vi "Climb_Motors.vi"(4 "Driver - Right Thumb":bool, 5 "Driver - Left Middle":bool, 6 "Driver - Left Thumb":bool, 7 "Driver - Right Middle":bool, 8 "Driver - Trigger":bool, 9 "Driver - Left Top left":bool, 10 "Driver - Right Top Right":bool) -> ()   [LabVIEW 2020]
uses:
  <vilib>/Rock Robotics/WPI/ThirdParty/Phoenix-LabVIEW/Motor Controller/Controls/CTRE_Phoenix_MotorControl_ControlMode.ctl
  <vilib>/Rock Robotics/Network Tables/NT Read String.vi
panel:
  in  "Traversal 1":dbl
  in  "Traversal 2":dbl
  in  "High 1":dbl
  in  "High 2":dbl
  in  "Mid 1":dbl=377500.0
  in  "Mid 2":dbl=377500.0
  in  "Low 1":dbl=150000.0
  in  "Low 2":dbl=150000.0
  in  "Low 4":dbl=150000.0
  in  "Low 3":dbl=150000.0
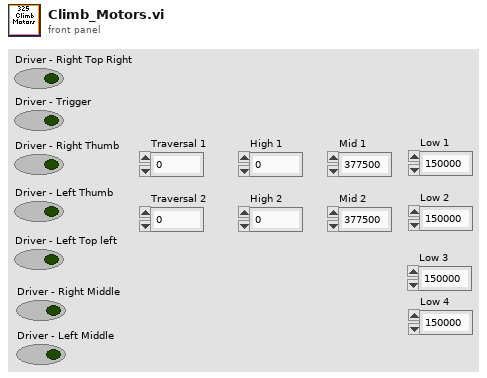
[diagram p1: front panel]
types:
  T1 = typedef "WPI_MotorControlDeviceRef.ctl" = cluster{"DeviceStatus":errorcluster, "Type":T2, "PWM":cluster{"PWM Channel":T3, "DeadBand":T4}, "CAN":cluster{"Device Number":u8, "SetOutput VI Ref":variant, "GetOutput VI Ref":variant, "Enable VI Ref":variant, "Disable VI Ref":variant, "Data":variant}, "Invert":bool, "DIO PWM":cluster{"PWM \"Enable\" Channel":T3, "DIOChannel":T5, "PWM Rate":dbl}}
  T2 = typedef "WPI_MotorControlType.ctl" = enum16{"PWM", "CAN", "DIO PWM"}
  T3 = typedef "FPGA_DIOPWMChannel.ctl" = enum8{"PWM 0", "PWM 1", "PWM 2", "PWM 3", "PWM 4", "PWM 5", "PWM 6", "PWM 7", "PWM 8", "PWM 9", "PWM MXP 0", "PWM MXP 1", "PWM MXP 2", "PWM MXP 3", "PWM MXP 4", "PWM MXP 5", "PWM MXP 6", "PWM MXP 7", "PWM MXP 8", "PWM MXP 9", "Invalid"}
  T4 = typedef "WPI_PWMDeadband.ctl" = cluster{"Name":string, "maxPositivePwm":i32, "minPositivePwm":i32, "centerPwm":i32, "maxNegativePwm":i32, "minNegativePwm":i32, "angularRange":u16}
  T5 = typedef "FPGA_DIOChannel.ctl" = enum8{"DIO 0", "DIO 1", "DIO 2", "DIO 3", "DIO 4", "DIO 5", "DIO 6", "DIO 7", "DIO 8", "DIO 9", "DIO MXP 0", "DIO MXP 1", "DIO MXP 2", "DIO MXP 3", "DIO MXP 4", "DIO MXP 5", "DIO MXP 6", "DIO MXP 7", "DIO MXP 8", "DIO MXP 9", "DIO MXP 10", "DIO MXP 11", "DIO MXP 12", "DIO MXP 13", "DIO MXP 14", "DIO MXP 15", "SPI Port CS1", "SPI Port CS2", "SPI Port CS3", "SPI Port MISO", "SPI Port MOSI", "Invalid"}
  T6 = typedef "CTRE_Phoenix_MotorControl_ControlMode.ctl" = u16
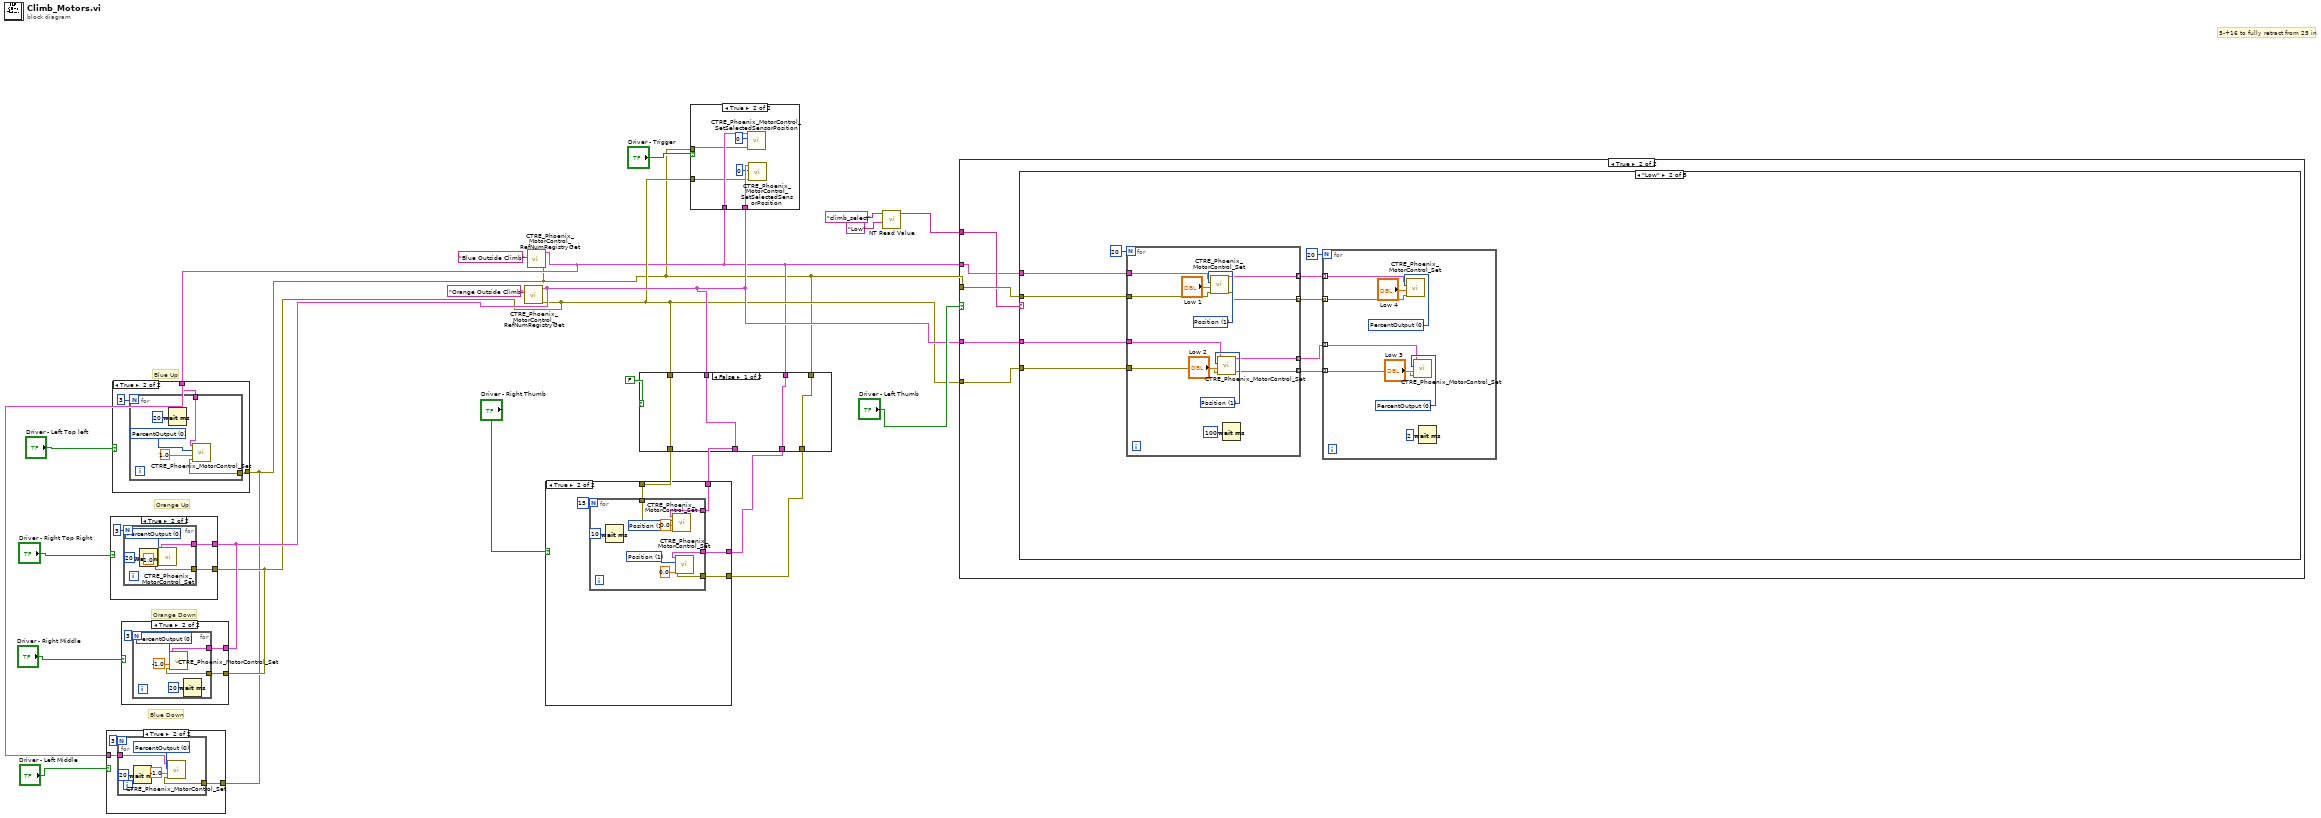
[diagram p0: block diagram]
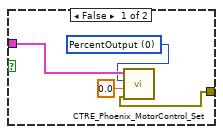
[diagram p2: hidden frame]
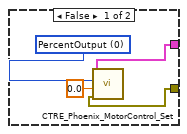
[diagram p3: hidden frame]
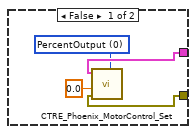
[diagram p4: hidden frame]
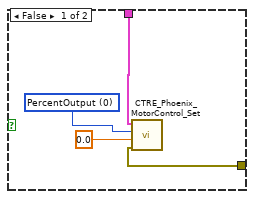
[diagram p5: hidden frame]
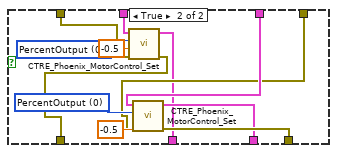
[diagram p6: hidden frame]
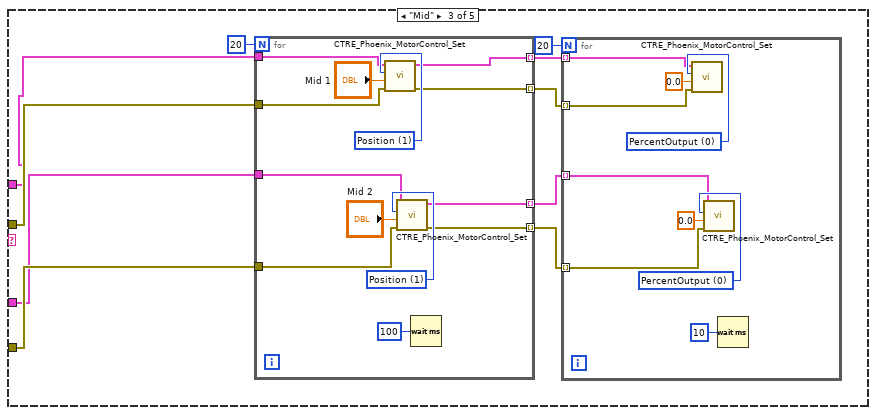
[diagram p10: hidden frame]
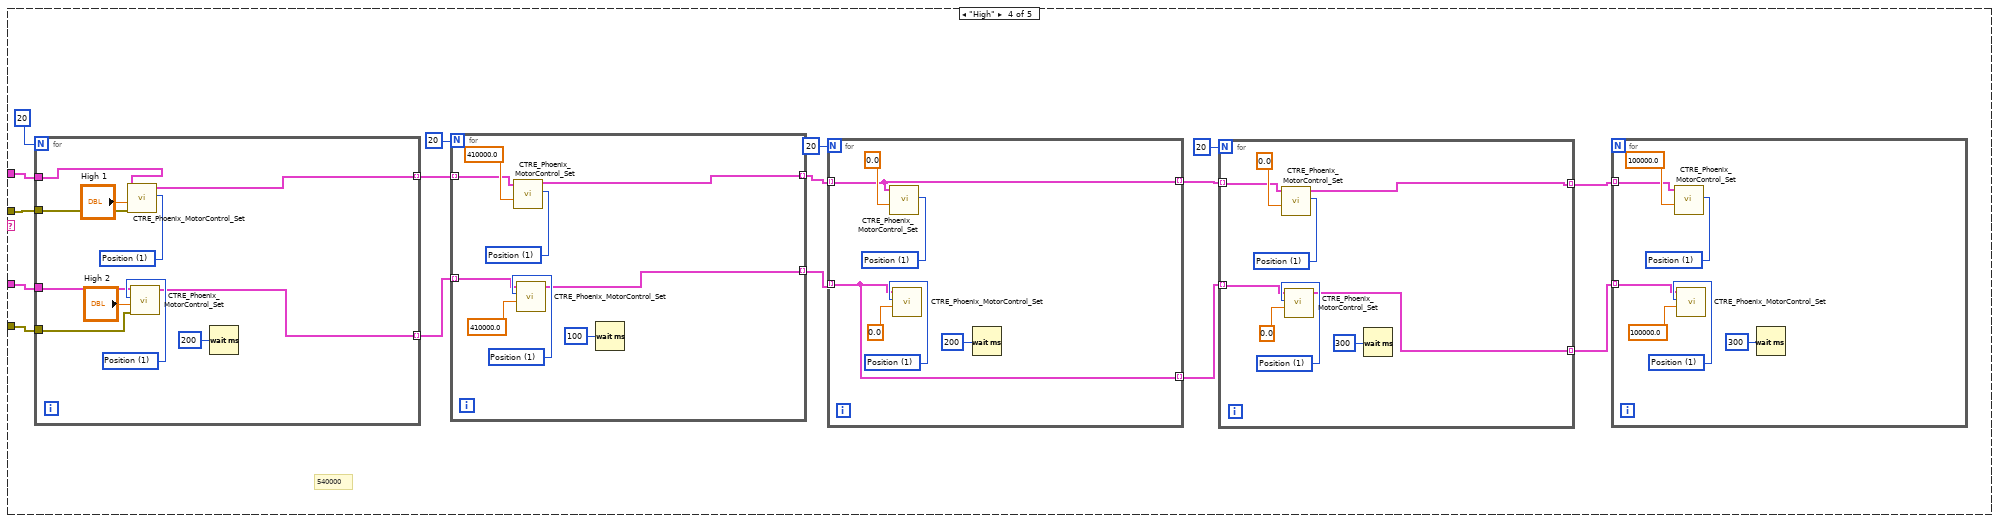
[diagram p11: hidden frame]
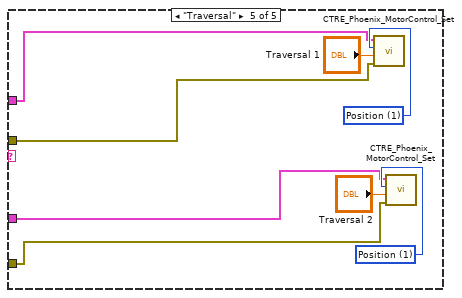
[diagram p12: hidden frame]
diagram:
  # "Blue Down"
  # "Orange Down"
  # "Orange Up"
  # "Blue Up"
  # "5-+16 to fully retract from 25 in"
  n1 = call <vilib>:"CTRE_Phoenix_MotorControl_RefNumRegistryGet.vi"("refnum name"="Orange Outside Climb") -> ("error out"=w4:errorcluster, "PhoenixMotorControlDevRef"=w5:T1)  [unwired: 9 in]
  n2 = case shown="True" "Driver - Right Top Right" {
    tunnel: w5 -> [w23 w28]
    tunnel: w4 -> [w24 w27]
    frame False {
      w22 = T6 0 items=["PercentOutput"=0, "Position"=1, "Velocity"=2, "Current"=3, "Follower"=5, "MotionProfile"=6, "MotionMagic"=7, "MotionProfileArc"=10, "Disabled"=15] ("Control Mode")
      n3 = call <vilib>:"CTRE_Phoenix_MotorControl_Set.vi"("error in (no error)"=w24, "Output"=0.0, "Control Mode"=w22, "PhoenixMotorControlDevRef"=w23) -> ()  [unwired: 6 in, 2 out]
    }
    frame True {
      n4 = for {
        N: 3 -> [_]
        tunnel: w28 -> [w31]
        tunnel: w27 -> [w30]
        w33 = T6 0 items=["PercentOutput"=0, "Position"=1, "Velocity"=2, "Current"=3, "Follower"=5, "MotionProfile"=6, "MotionMagic"=7, "MotionProfileArc"=10, "Disabled"=15] ("Control Mode")
        n5 = Wait (ms)(milliseconds to wait=u32 20) -> ()  [unwired: 1 out]
        n6 = call <vilib>:"CTRE_Phoenix_MotorControl_Set.vi"("error in (no error)"=w30, "Output"=1.0, "Control Mode"=w33, "PhoenixMotorControlDevRef"=w31) -> ()  [unwired: 6 in, 2 out]
      }
    }
  }
  n7 = case shown="True" "Driver - Right Middle" {
    tunnel: w5 -> [w35 w40]
    tunnel: w4 -> [w36 w39]
    frame False {
      w34 = T6 0 items=["PercentOutput"=0, "Position"=1, "Velocity"=2, "Current"=3, "Follower"=5, "MotionProfile"=6, "MotionMagic"=7, "MotionProfileArc"=10, "Disabled"=15] ("Control Mode")
      n8 = call <vilib>:"CTRE_Phoenix_MotorControl_Set.vi"("error in (no error)"=w36, "Output"=0.0, "Control Mode"=w34, "PhoenixMotorControlDevRef"=w35) -> ()  [unwired: 6 in, 2 out]
    }
    frame True {
      n9 = for {
        N: 3 -> [_]
        tunnel: w40 -> [w43]
        tunnel: w39 -> [w42]
        w45 = T6 0 items=["PercentOutput"=0, "Position"=1, "Velocity"=2, "Current"=3, "Follower"=5, "MotionProfile"=6, "MotionMagic"=7, "MotionProfileArc"=10, "Disabled"=15] ("Control Mode")
        n10 = call <vilib>:"CTRE_Phoenix_MotorControl_Set.vi"("error in (no error)"=w42, "Output"=-1.0, "Control Mode"=w45, "PhoenixMotorControlDevRef"=w43) -> ()  [unwired: 6 in, 2 out]
        n11 = Wait (ms)(milliseconds to wait=u32 20) -> ()  [unwired: 1 out]
      }
    }
  }
  n12 = call <vilib>:"CTRE_Phoenix_MotorControl_RefNumRegistryGet.vi"("refnum name"="Blue Outside Climb") -> ("error out"=w2:errorcluster, "PhoenixMotorControlDevRef"=w3:T1)  [unwired: 9 in]
  n13 = case shown="True" "Driver - Left Middle" {
    tunnel: w3 -> [w47 w52]
    tunnel: w2 -> [w48 w51]
    frame False {
      w46 = T6 0 items=["PercentOutput"=0, "Position"=1, "Velocity"=2, "Current"=3, "Follower"=5, "MotionProfile"=6, "MotionMagic"=7, "MotionProfileArc"=10, "Disabled"=15] ("Control Mode")
      n14 = call <vilib>:"CTRE_Phoenix_MotorControl_Set.vi"("error in (no error)"=w48, "Output"=0.0, "Control Mode"=w46, "PhoenixMotorControlDevRef"=w47) -> ()  [unwired: 6 in, 2 out]
    }
    frame True {
      n15 = for {
        N: 3 -> [_]
        tunnel: w52 -> [w55]
        tunnel: w51 -> [w54]
        w57 = T6 0 items=["PercentOutput"=0, "Position"=1, "Velocity"=2, "Current"=3, "Follower"=5, "MotionProfile"=6, "MotionMagic"=7, "MotionProfileArc"=10, "Disabled"=15] ("Control Mode")
        n16 = Wait (ms)(milliseconds to wait=u32 20) -> ()  [unwired: 1 out]
        n17 = call <vilib>:"CTRE_Phoenix_MotorControl_Set.vi"("error in (no error)"=w54, "Output"=-1.0, "Control Mode"=w57, "PhoenixMotorControlDevRef"=w55) -> ()  [unwired: 6 in, 2 out]
      }
    }
  }
  n18 = case shown="True" "Driver - Left Top left" {
    tunnel: w3 -> [w58 w64]
    tunnel: w2 -> [w59 w63]
    frame False {
      w60 = T6 0 items=["PercentOutput"=0, "Position"=1, "Velocity"=2, "Current"=3, "Follower"=5, "MotionProfile"=6, "MotionMagic"=7, "MotionProfileArc"=10, "Disabled"=15] ("Control Mode")
      n19 = call <vilib>:"CTRE_Phoenix_MotorControl_Set.vi"("error in (no error)"=w59, "Output"=0.0, "Control Mode"=w60, "PhoenixMotorControlDevRef"=w58) -> ()  [unwired: 6 in, 2 out]
    }
    frame True {
      n20 = for {
        N: 3 -> [_]
        tunnel: w64 -> [w67]
        tunnel: w63 -> [w66]
        w68 = T6 0 items=["PercentOutput"=0, "Position"=1, "Velocity"=2, "Current"=3, "Follower"=5, "MotionProfile"=6, "MotionMagic"=7, "MotionProfileArc"=10, "Disabled"=15] ("Control Mode")
        n21 = Wait (ms)(milliseconds to wait=u32 20) -> ()  [unwired: 1 out]
        n22 = call <vilib>:"CTRE_Phoenix_MotorControl_Set.vi"("error in (no error)"=w66, "Output"=1.0, "Control Mode"=w68, "PhoenixMotorControlDevRef"=w67) -> ()  [unwired: 6 in, 2 out]
      }
    }
  }
  n23 = case shown="False" FALSE {
    tunnel: w4 -> [w73 w80]
    tunnel: [w73 w74] -> w13
    tunnel: w5 -> [w72 w81]
    tunnel: [w72 w75] -> w12
    tunnel: [w71 w76] -> w11
    tunnel: w3 -> [w71 w79]
    tunnel: [w70 w77] -> w10
    tunnel: w2 -> [w70 w78]
    frame False {
    }
    frame True {
      w84 = T6 0 items=["PercentOutput"=0, "Position"=1, "Velocity"=2, "Current"=3, "Follower"=5, "MotionProfile"=6, "MotionMagic"=7, "MotionProfileArc"=10, "Disabled"=15] ("Control Mode")
      w85 = T6 0 items=["PercentOutput"=0, "Position"=1, "Velocity"=2, "Current"=3, "Follower"=5, "MotionProfile"=6, "MotionMagic"=7, "MotionProfileArc"=10, "Disabled"=15] ("Control Mode")
      n24 = call <vilib>:"CTRE_Phoenix_MotorControl_Set.vi"("error in (no error)"=w80, "Output"=-0.5, "Control Mode"=w84, "PhoenixMotorControlDevRef"=w81) -> ("error out"=w74:errorcluster, "PhoenixMotorControlDevRef"=w75:T1)  [unwired: 6 in]
      n25 = call <vilib>:"CTRE_Phoenix_MotorControl_Set.vi"("error in (no error)"=w78, "Output"=-0.5, "Control Mode"=w85, "PhoenixMotorControlDevRef"=w79) -> ("error out"=w77:errorcluster, "PhoenixMotorControlDevRef"=w76:T1)  [unwired: 6 in]
    }
  }
  n26 = case shown="True" "Driver - Right Thumb" {
    tunnel: w12 -> [_ w90]
    tunnel: w13 -> [_ w89]
    tunnel: w11 -> [_ w88]
    tunnel: w10 -> [_ w87]
    frame False {
    }
    frame True {
      n27 = for {
        N: 15 -> [_]
        tunnel: w90 -> [w95]
        tunnel: w89 -> [w94]
        tunnel: w88 -> [w93]
        tunnel: w87 -> [w92]
        w98 = T6 1 items=["PercentOutput"=0, "Position"=1, "Velocity"=2, "Current"=3, "Follower"=5, "MotionProfile"=6, "MotionMagic"=7, "MotionProfileArc"=10, "Disabled"=15] ("Control Mode")
        w99 = T6 1 items=["PercentOutput"=0, "Position"=1, "Velocity"=2, "Current"=3, "Follower"=5, "MotionProfile"=6, "MotionMagic"=7, "MotionProfileArc"=10, "Disabled"=15] ("Control Mode")
        n28 = Wait (ms)(milliseconds to wait=u32 10) -> ()  [unwired: 1 out]
        n29 = call <vilib>:"CTRE_Phoenix_MotorControl_Set.vi"("error in (no error)"=w94, "Output"=0.0, "Control Mode"=w98, "PhoenixMotorControlDevRef"=w95) -> ()  [unwired: 6 in, 2 out]
        n30 = call <vilib>:"CTRE_Phoenix_MotorControl_Set.vi"("error in (no error)"=w92, "Output"=0.0, "Control Mode"=w99, "PhoenixMotorControlDevRef"=w93) -> ()  [unwired: 6 in, 2 out]
      }
    }
  }
  n31 = case shown="True" "Driver - Trigger" {
    tunnel: w3 -> [_ w105]
    tunnel: w2 -> [_ w104]
    tunnel: w5 -> [_ w103]
    tunnel: w4 -> [_ w102]
    frame False {
    }
    frame True {
      n32 = call <vilib>:"CTRE_Phoenix_MotorControl_SetSelectedSensorPosition.vi"("error in (no error)"=w104, "New Sensor Position"=0, "PhoenixMotorControlDevRef"=w105) -> ()  [unwired: 7 in, 2 out]
      n33 = call <vilib>:"CTRE_Phoenix_MotorControl_SetSelectedSensorPosition.vi"("error in (no error)"=w102, "New Sensor Position"=0, "PhoenixMotorControlDevRef"=w103) -> ()  [unwired: 7 in, 2 out]
    }
  }
  n34 = call-poly <vilib>:"NT Read Value.vi"("Default Value"="Low", "Name"="climb_select") -> ("String"=w16:string)  [unwired: 8 in, 1 out]
  n35 = case shown="True" "Driver - Left Thumb" {
    tunnel: w3 -> [_ w106]
    tunnel: w2 -> [_ w110]
    tunnel: w5 -> [_ w109]
    tunnel: w4 -> [_ w108]
    tunnel: w16 -> [_ w107]
    frame False {
    }
    frame True {
      n36 = case shown="\"Low\"" w107 {
        tunnel: w110 -> [_ w120 w152 w190 w237]
        tunnel: w109 -> [_ w119 w150 w189 w236]
        tunnel: w108 -> [_ w118 w151 w188 w235]
        tunnel: w106 -> [_ w117 w149 w187 w234]
        frame Default {
        }
        frame "Low" {
          n37 = for {
            N: 20 -> [_]
            tunnel: w120 -> [w140]
            tunnel: w119 -> [w137]
            tunnel: w118 -> [w136]
            tunnel: w117 -> [w135]
            tunnel: [w133] -> w115 mode=indexing
            tunnel: [w132] -> w114 mode=indexing
            tunnel: [w131] -> w113 mode=indexing
            tunnel: [w130] -> w112 mode=indexing
            w138 = T6 1 items=["PercentOutput"=0, "Position"=1, "Velocity"=2, "Current"=3, "Follower"=5, "MotionProfile"=6, "MotionMagic"=7, "MotionProfileArc"=10, "Disabled"=15] ("Control Mode")
            w141 = T6 1 items=["PercentOutput"=0, "Position"=1, "Velocity"=2, "Current"=3, "Follower"=5, "MotionProfile"=6, "MotionMagic"=7, "MotionProfileArc"=10, "Disabled"=15] ("Control Mode")
            n38 = call <vilib>:"CTRE_Phoenix_MotorControl_Set.vi"("error in (no error)"=w140, "Output"="Low 1", "Control Mode"=w141, "PhoenixMotorControlDevRef"=w135) -> ("error out"=w132:errorcluster, "PhoenixMotorControlDevRef"=w133:T1)  [unwired: 6 in]
            n39 = call <vilib>:"CTRE_Phoenix_MotorControl_Set.vi"("error in (no error)"=w136, "Output"="Low 2", "Control Mode"=w138, "PhoenixMotorControlDevRef"=w137) -> ("error out"=w130:errorcluster, "PhoenixMotorControlDevRef"=w131:T1)  [unwired: 6 in]
            n40 = Wait (ms)(milliseconds to wait=u32 100) -> ()  [unwired: 1 out]
          }
          n41 = for {
            N: 20 -> [_]
            tunnel: w114 -> [w127] mode=indexing
            tunnel: w113 -> [w124] mode=indexing
            tunnel: w112 -> [w123] mode=indexing
            tunnel: w115 -> [w122] mode=indexing
            w125 = T6 0 items=["PercentOutput"=0, "Position"=1, "Velocity"=2, "Current"=3, "Follower"=5, "MotionProfile"=6, "MotionMagic"=7, "MotionProfileArc"=10, "Disabled"=15] ("Control Mode")
            w128 = T6 0 items=["PercentOutput"=0, "Position"=1, "Velocity"=2, "Current"=3, "Follower"=5, "MotionProfile"=6, "MotionMagic"=7, "MotionProfileArc"=10, "Disabled"=15] ("Control Mode")
            n42 = call <vilib>:"CTRE_Phoenix_MotorControl_Set.vi"("error in (no error)"=w127, "Output"="Low 4", "Control Mode"=w128, "PhoenixMotorControlDevRef"=w122) -> ()  [unwired: 6 in, 2 out]
            n43 = call <vilib>:"CTRE_Phoenix_MotorControl_Set.vi"("error in (no error)"=w123, "Output"="Low 3", "Control Mode"=w125, "PhoenixMotorControlDevRef"=w124) -> ()  [unwired: 6 in, 2 out]
            n44 = Wait (ms)(milliseconds to wait=u32 2) -> ()  [unwired: 1 out]
          }
        }
        frame "Mid" {
          n45 = for {
            N: 20 -> [_]
            tunnel: w152 -> [w170]
            tunnel: w151 -> [w169]
            tunnel: w150 -> [w168]
            tunnel: w149 -> [w167]
            tunnel: [w165] -> w147 mode=indexing
            tunnel: [w164] -> w146 mode=indexing
            tunnel: [w163] -> w145 mode=indexing
            tunnel: [w162] -> w144 mode=indexing
            w171 = T6 1 items=["PercentOutput"=0, "Position"=1, "Velocity"=2, "Current"=3, "Follower"=5, "MotionProfile"=6, "MotionMagic"=7, "MotionProfileArc"=10, "Disabled"=15] ("Control Mode")
            w173 = T6 1 items=["PercentOutput"=0, "Position"=1, "Velocity"=2, "Current"=3, "Follower"=5, "MotionProfile"=6, "MotionMagic"=7, "MotionProfileArc"=10, "Disabled"=15] ("Control Mode")
            n46 = call <vilib>:"CTRE_Phoenix_MotorControl_Set.vi"("error in (no error)"=w170, "Output"="Mid 1", "Control Mode"=w173, "PhoenixMotorControlDevRef"=w167) -> ("error out"=w163:errorcluster, "PhoenixMotorControlDevRef"=w162:T1)  [unwired: 6 in]
            n47 = call <vilib>:"CTRE_Phoenix_MotorControl_Set.vi"("error in (no error)"=w169, "Output"="Mid 2", "Control Mode"=w171, "PhoenixMotorControlDevRef"=w168) -> ("error out"=w165:errorcluster, "PhoenixMotorControlDevRef"=w164:T1)  [unwired: 6 in]
            n48 = Wait (ms)(milliseconds to wait=u32 100) -> ()  [unwired: 1 out]
          }
          n49 = for {
            N: 20 -> [_]
            tunnel: w145 -> [w159] mode=indexing
            tunnel: w147 -> [w158] mode=indexing
            tunnel: w146 -> [w157] mode=indexing
            tunnel: w144 -> [w156] mode=indexing
            w160 = T6 0 items=["PercentOutput"=0, "Position"=1, "Velocity"=2, "Current"=3, "Follower"=5, "MotionProfile"=6, "MotionMagic"=7, "MotionProfileArc"=10, "Disabled"=15] ("Control Mode")
            w161 = T6 0 items=["PercentOutput"=0, "Position"=1, "Velocity"=2, "Current"=3, "Follower"=5, "MotionProfile"=6, "MotionMagic"=7, "MotionProfileArc"=10, "Disabled"=15] ("Control Mode")
            n50 = call <vilib>:"CTRE_Phoenix_MotorControl_Set.vi"("error in (no error)"=w159, "Output"=0.0, "Control Mode"=w161, "PhoenixMotorControlDevRef"=w156) -> ()  [unwired: 6 in, 2 out]
            n51 = call <vilib>:"CTRE_Phoenix_MotorControl_Set.vi"("error in (no error)"=w158, "Output"=0.0, "Control Mode"=w160, "PhoenixMotorControlDevRef"=w157) -> ()  [unwired: 6 in, 2 out]
            n52 = Wait (ms)(milliseconds to wait=u32 10) -> ()  [unwired: 1 out]
          }
        }
        frame "High" {
          # "540000"
          n53 = for {
            N: 20 -> [_]
            tunnel: w190 -> [w229]
            tunnel: w189 -> [w228]
            tunnel: w188 -> [w227]
            tunnel: w187 -> [w225]
            tunnel: [w224] -> w185 mode=indexing
            tunnel: [w223] -> w184 mode=indexing
            w230 = T6 1 items=["PercentOutput"=0, "Position"=1, "Velocity"=2, "Current"=3, "Follower"=5, "MotionProfile"=6, "MotionMagic"=7, "MotionProfileArc"=10, "Disabled"=15] ("Control Mode")
            w232 = T6 1 items=["PercentOutput"=0, "Position"=1, "Velocity"=2, "Current"=3, "Follower"=5, "MotionProfile"=6, "MotionMagic"=7, "MotionProfileArc"=10, "Disabled"=15] ("Control Mode")
            n54 = call <vilib>:"CTRE_Phoenix_MotorControl_Set.vi"("error in (no error)"=w229, "Output"="High 1", "Control Mode"=w232, "PhoenixMotorControlDevRef"=w225) -> ("PhoenixMotorControlDevRef"=w224:T1)  [unwired: 6 in, 1 out]
            n55 = call <vilib>:"CTRE_Phoenix_MotorControl_Set.vi"("error in (no error)"=w227, "Output"="High 2", "Control Mode"=w230, "PhoenixMotorControlDevRef"=w228) -> ("PhoenixMotorControlDevRef"=w223:T1)  [unwired: 6 in, 1 out]
            n56 = Wait (ms)(milliseconds to wait=u32 200) -> ()  [unwired: 1 out]
          }
          n57 = for {
            N: 20 -> [_]
            tunnel: w185 -> [w217] mode=indexing
            tunnel: w184 -> [w216] mode=indexing
            tunnel: [w215] -> w182 mode=indexing
            tunnel: [w214] -> w181 mode=indexing
            w219 = T6 1 items=["PercentOutput"=0, "Position"=1, "Velocity"=2, "Current"=3, "Follower"=5, "MotionProfile"=6, "MotionMagic"=7, "MotionProfileArc"=10, "Disabled"=15] ("Control Mode")
            w221 = T6 1 items=["PercentOutput"=0, "Position"=1, "Velocity"=2, "Current"=3, "Follower"=5, "MotionProfile"=6, "MotionMagic"=7, "MotionProfileArc"=10, "Disabled"=15] ("Control Mode")
            n58 = call <vilib>:"CTRE_Phoenix_MotorControl_Set.vi"("Output"=410000.0 ("High 8"), "Control Mode"=w221, "PhoenixMotorControlDevRef"=w217) -> ("PhoenixMotorControlDevRef"=w215:T1)  [unwired: 7 in, 1 out]
            n59 = call <vilib>:"CTRE_Phoenix_MotorControl_Set.vi"("Output"=410000.0 ("High 7"), "Control Mode"=w219, "PhoenixMotorControlDevRef"=w216) -> ("PhoenixMotorControlDevRef"=w214:T1)  [unwired: 7 in, 1 out]
            n60 = Wait (ms)(milliseconds to wait=u32 100) -> ()  [unwired: 1 out]
          }
          n61 = for {
            N: 20 -> [_]
            tunnel: w182 -> [w208] mode=indexing
            tunnel: w181 -> [w207] mode=indexing
            tunnel: [w208] -> w178 mode=indexing
            tunnel: [w207] -> w177 mode=indexing
            w210 = T6 1 items=["PercentOutput"=0, "Position"=1, "Velocity"=2, "Current"=3, "Follower"=5, "MotionProfile"=6, "MotionMagic"=7, "MotionProfileArc"=10, "Disabled"=15] ("Control Mode")
            w212 = T6 1 items=["PercentOutput"=0, "Position"=1, "Velocity"=2, "Current"=3, "Follower"=5, "MotionProfile"=6, "MotionMagic"=7, "MotionProfileArc"=10, "Disabled"=15] ("Control Mode")
            n62 = call <vilib>:"CTRE_Phoenix_MotorControl_Set.vi"("Output"=0.0 ("High 8"), "Control Mode"=w212, "PhoenixMotorControlDevRef"=w208) -> ()  [unwired: 7 in, 2 out]
            n63 = call <vilib>:"CTRE_Phoenix_MotorControl_Set.vi"("Output"=0.0 ("High 7"), "Control Mode"=w210, "PhoenixMotorControlDevRef"=w207) -> ()  [unwired: 7 in, 2 out]
            n64 = Wait (ms)(milliseconds to wait=u32 200) -> ()  [unwired: 1 out]
          }
          n65 = for {
            N: 20 -> [_]
            tunnel: w178 -> [w201] mode=indexing
            tunnel: w177 -> [w200] mode=indexing
            tunnel: [w199] -> w176 mode=indexing
            tunnel: [w198] -> w175 mode=indexing
            w203 = T6 1 items=["PercentOutput"=0, "Position"=1, "Velocity"=2, "Current"=3, "Follower"=5, "MotionProfile"=6, "MotionMagic"=7, "MotionProfileArc"=10, "Disabled"=15] ("Control Mode")
            w205 = T6 1 items=["PercentOutput"=0, "Position"=1, "Velocity"=2, "Current"=3, "Follower"=5, "MotionProfile"=6, "MotionMagic"=7, "MotionProfileArc"=10, "Disabled"=15] ("Control Mode")
            n66 = call <vilib>:"CTRE_Phoenix_MotorControl_Set.vi"("Output"=0.0 ("High 8"), "Control Mode"=w205, "PhoenixMotorControlDevRef"=w201) -> ("PhoenixMotorControlDevRef"=w199:T1)  [unwired: 7 in, 1 out]
            n67 = call <vilib>:"CTRE_Phoenix_MotorControl_Set.vi"("Output"=0.0 ("High 7"), "Control Mode"=w203, "PhoenixMotorControlDevRef"=w200) -> ("PhoenixMotorControlDevRef"=w198:T1)  [unwired: 7 in, 1 out]
            n68 = Wait (ms)(milliseconds to wait=u32 300) -> ()  [unwired: 1 out]
          }
          n69 = for {
            tunnel: w176 -> [w192] mode=indexing
            tunnel: w175 -> [w191] mode=indexing
            w194 = T6 1 items=["PercentOutput"=0, "Position"=1, "Velocity"=2, "Current"=3, "Follower"=5, "MotionProfile"=6, "MotionMagic"=7, "MotionProfileArc"=10, "Disabled"=15] ("Control Mode")
            w196 = T6 1 items=["PercentOutput"=0, "Position"=1, "Velocity"=2, "Current"=3, "Follower"=5, "MotionProfile"=6, "MotionMagic"=7, "MotionProfileArc"=10, "Disabled"=15] ("Control Mode")
            n70 = call <vilib>:"CTRE_Phoenix_MotorControl_Set.vi"("Output"=100000.0 ("High 8"), "Control Mode"=w196, "PhoenixMotorControlDevRef"=w192) -> ()  [unwired: 7 in, 2 out]
            n71 = call <vilib>:"CTRE_Phoenix_MotorControl_Set.vi"("Output"=100000.0 ("High 7"), "Control Mode"=w194, "PhoenixMotorControlDevRef"=w191) -> ()  [unwired: 7 in, 2 out]
            n72 = Wait (ms)(milliseconds to wait=u32 300) -> ()  [unwired: 1 out]
          }
        }
        frame "Traversal" {
          w238 = T6 1 items=["PercentOutput"=0, "Position"=1, "Velocity"=2, "Current"=3, "Follower"=5, "MotionProfile"=6, "MotionMagic"=7, "MotionProfileArc"=10, "Disabled"=15] ("Control Mode")
          w240 = T6 1 items=["PercentOutput"=0, "Position"=1, "Velocity"=2, "Current"=3, "Follower"=5, "MotionProfile"=6, "MotionMagic"=7, "MotionProfileArc"=10, "Disabled"=15] ("Control Mode")
          n73 = call <vilib>:"CTRE_Phoenix_MotorControl_Set.vi"("error in (no error)"=w237, "Output"="Traversal 1", "Control Mode"=w240, "PhoenixMotorControlDevRef"=w234) -> ()  [unwired: 6 in, 2 out]
          n74 = call <vilib>:"CTRE_Phoenix_MotorControl_Set.vi"("error in (no error)"=w235, "Output"="Traversal 2", "Control Mode"=w238, "PhoenixMotorControlDevRef"=w236) -> ()  [unwired: 6 in, 2 out]
        }
      }
    }
  }
